vi "Do.vi"(8 "error in (no error)":errorcluster, 10 "Actor in":refnum<class "Actor.lvclass">, 11 "open camera quick settings Msg":refnum<class "open camera quick settings Msg.lvclass">) -> (0 "error out":errorcluster, 2 "Actor out":refnum<class "Actor.lvclass">)   [LabVIEW 2014, in "IMAQdx Actor.lvlib" / "open camera quick settings Msg.lvclass"]
doc: "This VI delivers the message to the actor by calling the appropriate method(s) on the actor."
uses:
  open camera quick settings Msg.lvclass
  <vilib>/ActorFramework/Actor/Actor.lvclass
  IMAQdx Actor/IMAQdx Actor.lvclass
  open camera quick settings Msg.lvclass/open camera quick settings Msg.ctl
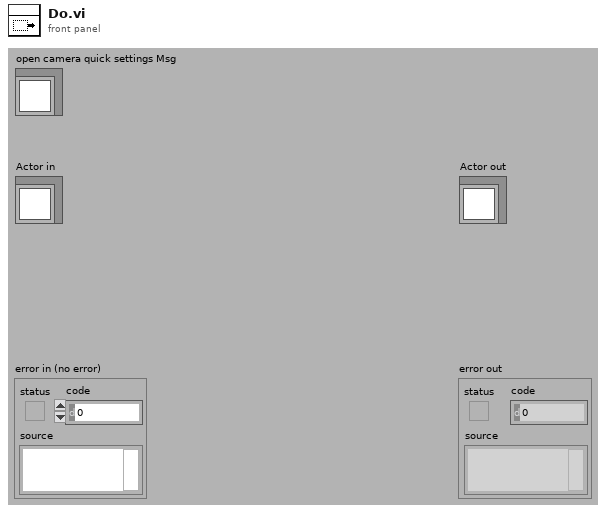
[diagram p1: front panel]
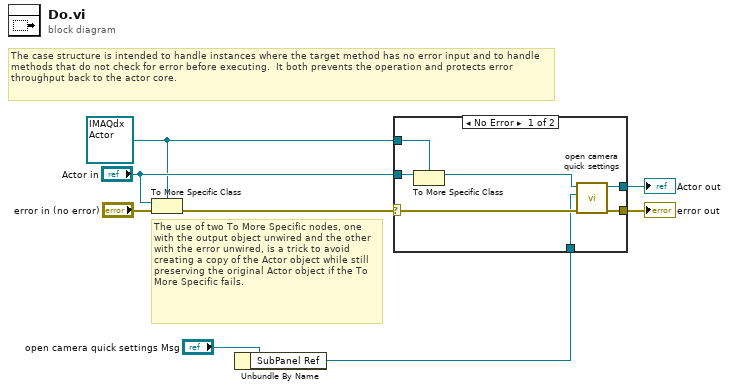
[diagram p0: block diagram]
diagram:
  w3 = refnum<class "IMAQdx Actor.lvclass"> refnum ("Actor in")
  # "The use of two To More Specific nodes, one with the output object unwired and the other with the error unwired, is a trick to avoid creating a copy of the Actor object while still preserving the original Actor object if the To More Specific fails."
  # "The case structure is intended to handle instances where the target method has no error input and to handle methods that do not check for error before executing.  It both prevents the operation and protects error throughput back to the actor core."
  n1 = To More Specific Class(target class=w3, reference="Actor in", error in="error in (no error)") -> (error out=w7:errorcluster)  [unwired: 1 out]
  n2 = Unbundle By Name("open camera quick settings Msg") -> ("SubPanel Ref"=w1:refnum<vi>)
  n3 = case shown="No Error" w7 {
    selector: w7 -> [w13 w17]
    tunnel: [w15 w17] -> w6
    tunnel: [w14 w16] -> w5
    tunnel: "Actor in" -> [w12 w16]
    tunnel: w3 -> [w11 _]
    tunnel: w1 -> [w9 _]
    frame No Error {
      n4 = To More Specific Class(target class=w11, reference=w12) -> (specific class reference=w10:refnum<class "IMAQdx Actor.lvclass">)  [unwired: 1 in, 1 out]
      n5 = call-dynamic "open camera quick settings.vi"("error in (no error)"=w13, "SubPanel Ref"=w9, "IMAQdx Actor in"=w10) -> ("error out"=w15:errorcluster, "IMAQdx Actor out"=w14:refnum<class "IMAQdx Actor.lvclass">)  [unwired: 7 in]
    }
    frame Error {
      # "If type check fails, pass the original object out again."
    }
  }
  "error out" <- w6
  "Actor out" <- w5
